vi "DriverStationGetCommands.vi"() -> ()   [LabVIEW 2019]
doc: "This VI receives instructions from the driver and manipulator controls, but only in certain robot modes. Specifically, these instructions are received while the robot is either \"running autonomously\" or in Super Test Mode. In all other robot modes, no instructions are received via the driver station. Instead they are output by the Autonomous Sequencer or completely disabled."
uses:
  refnums.vi
  dscommands.vi
  <vilib>/Rock Robotics/Network Tables/NT Read Boolean Array.vi
  dsdata.vi
  GRNF_Joystick.vi
  <vilib>/Rock Robotics/Network Tables/NT Read Boolean.vi
panel:
  in  "Buttons":bool[](array[boolean])=[FALSE, FALSE, FALSE, FALSE, FALSE, FALSE, FALSE, FALSE, FALSE, FALSE]
  in  "Right Trigger":dbl(slide) min=0.0 max=1.0 scale=0.0..1.0
  in  "Left Trigger":dbl(slide) min=0.0 max=1.0 step=0.1 scale=0.0..1.0
  in  "Right Joystick X":dbl(slide) scale=-1.0..1.0
  in  "Enable Joystick Control Override":bool
  in  "Joystick Left X":dbl(slide) scale=-1.0..1.0
  in  "Joystick Left Y":dbl(slide) scale=1.0..-1.0
  in  "Joystick Right Y":dbl(slide) scale=1.0..-1.0
  # "Left Thumbstick"
  # "Right Thumbstick"
  # "Driver A"
  # "Driver B"
  # "Driver X"
  # "Driver Y"
  # "Driver Left Bumper"
  # "Driver Right Bumper"
  # "Driver View"
  # "Driver Menu"
  # "Driver Left Joystick Button"
  # "Driver Right Joystick Button"
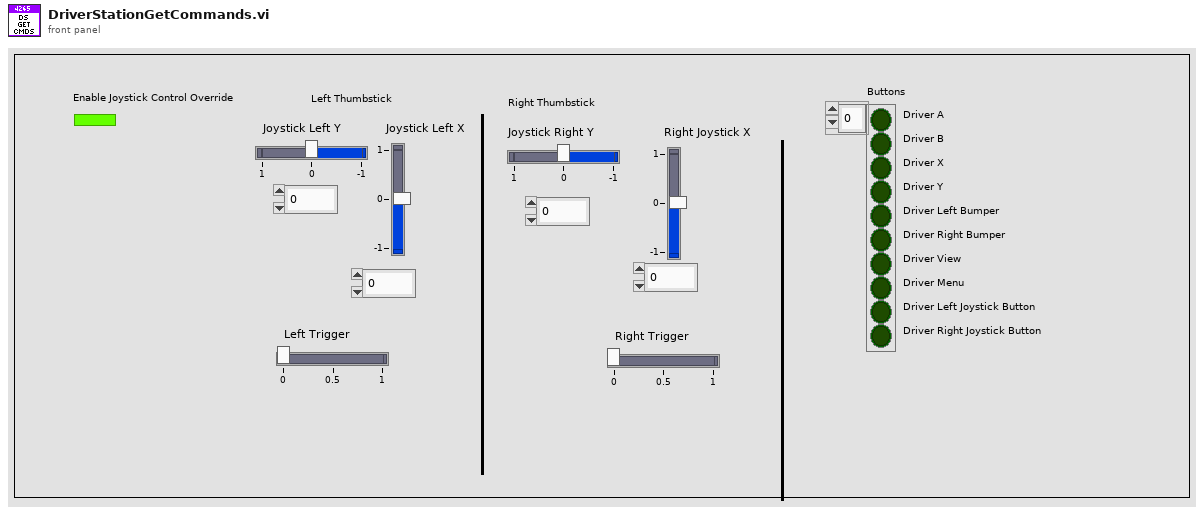
[diagram p1: front panel]
types:
  T1 = typedef "WPI_JoystickDevRef.ctl" = cluster{"Device":T2}
  T2 = typedef "WPI_JoystickDeviceEnum.ctl" = enum16{"USB 0", "USB 1", "USB 2", "USB 3", "USB 4", "USB 5"}
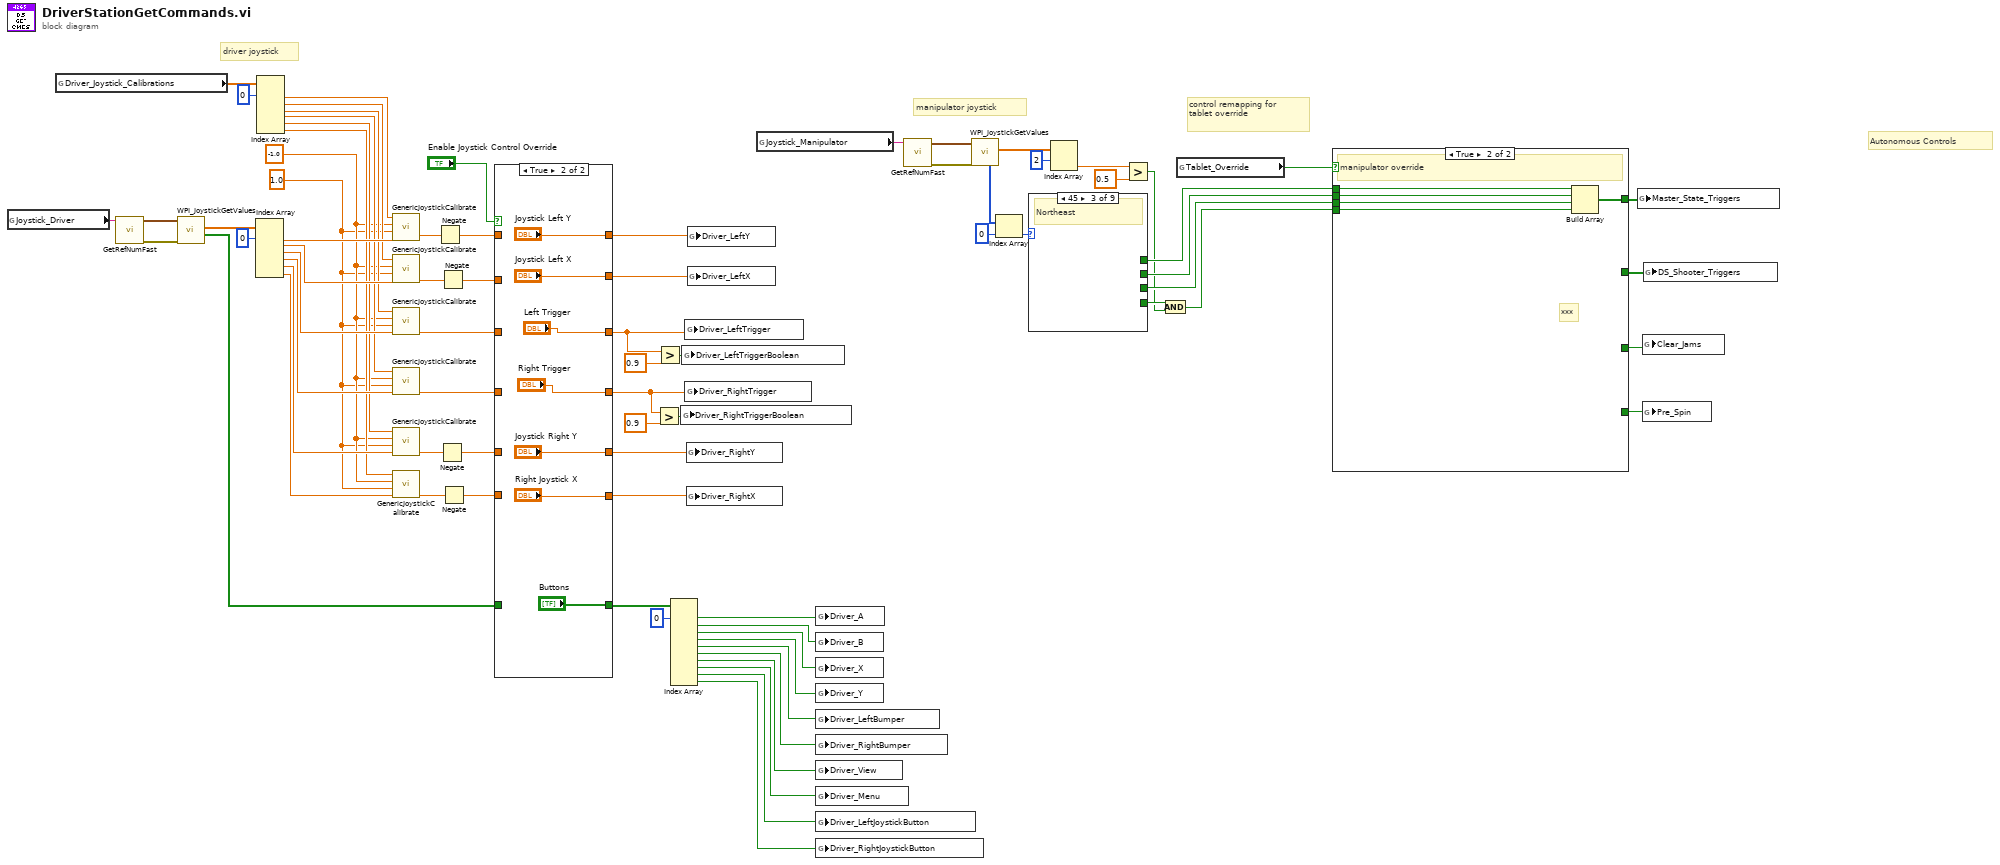
[diagram p0: block diagram]
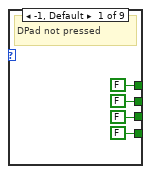
[diagram p3: hidden frame]
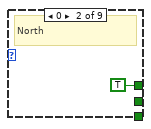
[diagram p4: hidden frame]
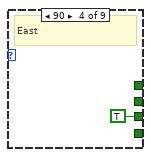
[diagram p5: hidden frame]
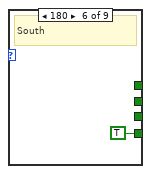
[diagram p7: hidden frame]
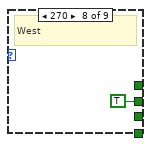
[diagram p9: hidden frame]
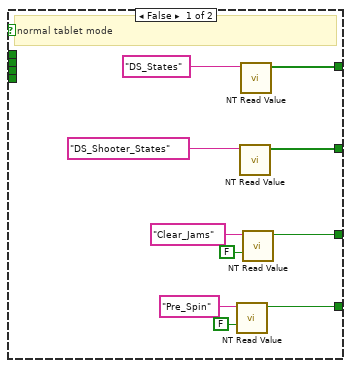
[diagram p11: hidden frame]
diagram:
  w22 = 1.0
  w23 = -1.0
  # "Autonomous Controls"
  # "control remapping for\ntablet override"
  # "manipulator joystick"
  # "driver joystick"
  n1 = global read "refnums.vi" "Joystick_Driver"() -> (w46:string)
  n2 = global read "dsdata.vi" "Driver_Joystick_Calibrations"() -> (w40:dbl[])
  n3 = call-poly "GetRefNumFast.vi"("RefNum Name"=w46) -> ("Error"=w47:errorcluster, "Device Reference"=w48:T1)  [unwired: 5 in]
  n4 = call <vilib>:"WPI_JoystickGetValues.vi"("error in (no error)"=w47, "JoystickDevRef"=w48) -> ("Buttons"=w4:bool[], "Axes"=w76:dbl[])  [unwired: 5 in, 3 out]
  n5 = Index Array(array=w76, index #1=0 ("index")) -> (element #1=w35:dbl, element #2=w34:dbl, element #3=w30:dbl, element #4=w31:dbl, element #5=w32:dbl, element #6=w33:dbl)  [unwired: 5 in]
  n6 = Index Array(array=w40, index #1=0 ("index")) -> (element #1=w24:dbl, element #2=w25:dbl, element #3=w26:dbl, element #4=w27:dbl, element #5=w28:dbl, element #6=w29:dbl)  [unwired: 5 in]
  n7 = call "GenericJoystickCalibrate.vi"("Raw Joystick Value"=w35, "Maximum"=w22, "Minimum"=w23, "Deadband"=w24) -> ("Scaled Joystick Value"=w39:dbl)  [unwired: 3 in]
  n8 = call "GenericJoystickCalibrate.vi"("Raw Joystick Value"=w34, "Maximum"=w22, "Minimum"=w23, "Deadband"=w25) -> ("Scaled Joystick Value"=w38:dbl)  [unwired: 3 in]
  n9 = call "GenericJoystickCalibrate.vi"("Raw Joystick Value"=w30, "Maximum"=w22, "Minimum"=w23, "Deadband"=w26) -> ("Scaled Joystick Value"=w16:dbl)  [unwired: 3 in]
  n10 = call "GenericJoystickCalibrate.vi"("Raw Joystick Value"=w31, "Maximum"=w22, "Minimum"=w23, "Deadband"=w27) -> ("Scaled Joystick Value"=w10:dbl)  [unwired: 3 in]
  n11 = call "GenericJoystickCalibrate.vi"("Raw Joystick Value"=w32, "Maximum"=w22, "Minimum"=w23, "Deadband"=w28) -> ("Scaled Joystick Value"=w37:dbl)  [unwired: 3 in]
  n12 = call "GenericJoystickCalibrate.vi"("Raw Joystick Value"=w33, "Maximum"=w22, "Minimum"=w23, "Deadband"=w29) -> ("Scaled Joystick Value"=w36:dbl)  [unwired: 3 in]
  n13 = Negate(x=w39) -> (-x=w19:dbl)
  n14 = Negate(x=w37) -> (-x=w7:dbl)
  n15 = Negate(x=w38) -> (-x=w18:dbl)
  n16 = Negate(x=w36) -> (-x=w6:dbl)
  n17 = case shown="True" "Enable Joystick Control Override" {
    tunnel: w16 -> [w81 _]
    tunnel: [w83 "Joystick Left Y"] -> w20
    tunnel: w19 -> [w83 _]
    tunnel: [w82 "Joystick Left X"] -> w17
    tunnel: w18 -> [w82 _]
    tunnel: [w81 "Left Trigger"] -> w11
    tunnel: w10 -> [w80 _]
    tunnel: [w80 "Right Trigger"] -> w9
    tunnel: [w79 "Joystick Right Y"] -> w8
    tunnel: w7 -> [w79 _]
    tunnel: [w78 "Right Joystick X"] -> w5
    tunnel: w6 -> [w78 _]
    tunnel: w4 -> [w77 _]
    tunnel: [w77 "Buttons"] -> w3
    frame False {
    }
    frame True {
    }
  }
  n18 = Greater?(x=w9, y=0.9) -> (0:w13:bool)
  n19 = Greater?(x=w11, y=0.9) -> (0:w12:bool)
  n20 = Index Array(array=w3, index #1=0 ("index")) -> (element #1=w73:bool, element #2=w72:bool, element #3=w71:bool, element #4=w70:bool, element #5=w69:bool, element #6=w68:bool, element #7=w67:bool, element #8=w66:bool, element #9=w65:bool, element #10=w64:bool)  [unwired: 9 in]
  n21 = global write "dscommands.vi" "Driver_RightTriggerBoolean"(w13) -> ()
  n22 = global write "dscommands.vi" "Driver_LeftTriggerBoolean"(w12) -> ()
  n23 = global write "dscommands.vi" "Driver_LeftTrigger"(w11) -> ()
  n24 = global write "dscommands.vi" "Driver_RightTrigger"(w9) -> ()
  n25 = global write "dscommands.vi" "Driver_RightY"(w8) -> ()
  n26 = global write "dscommands.vi" "Driver_RightX"(w5) -> ()
  n27 = global write "dscommands.vi" "Driver_LeftY"(w20) -> ()
  n28 = global write "dscommands.vi" "Driver_LeftX"(w17) -> ()
  n29 = global read "refnums.vi" "Joystick_Manipulator"() -> (w43:string)
  n30 = global write "dscommands.vi" "Driver_A"(w73) -> ()
  n31 = global write "dscommands.vi" "Driver_B"(w72) -> ()
  n32 = global write "dscommands.vi" "Driver_X"(w71) -> ()
  n33 = global write "dscommands.vi" "Driver_Y"(w70) -> ()
  n34 = global write "dscommands.vi" "Driver_LeftBumper"(w69) -> ()
  n35 = global write "dscommands.vi" "Driver_RightBumper"(w68) -> ()
  n36 = global write "dscommands.vi" "Driver_View"(w67) -> ()
  n37 = global write "dscommands.vi" "Driver_Menu"(w66) -> ()
  n38 = global write "dscommands.vi" "Driver_LeftJoystickButton"(w65) -> ()
  n39 = global write "dscommands.vi" "Driver_RightJoystickButton"(w64) -> ()
  n40 = call-poly "GetRefNumFast.vi"("RefNum Name"=w43) -> ("Error"=w44:errorcluster, "Device Reference"=w45:T1)  [unwired: 5 in]
  n41 = call <vilib>:"WPI_JoystickGetValues.vi"("error in (no error)"=w44, "JoystickDevRef"=w45) -> ("Axes"=w63:dbl[], "POVs"=w56:i16[])  [unwired: 5 in, 3 out]
  n42 = Index Array(array=w56, index=0) -> (element=w57:i16)
  n43 = case shown="45" w57 {
    tunnel: [FALSE TRUE _ _ _ _ _ _ _] -> w55
    tunnel: [FALSE _ _ _ _ _ _ TRUE _] -> w54
    tunnel: [FALSE _ _ TRUE _ _ _ _ _] -> w53
    tunnel: [FALSE _ _ _ _ TRUE _ _ _] -> w52
    frame -1, Default {
      # "DPad not pressed"
    }
    frame 0 {
      # "North"
    }
    frame 45 {
      # "Northeast"
    }
    frame 90 {
      # "East"
    }
    frame 135 {
      # "Southeast"
    }
    frame 180 {
      # "South"
    }
    frame 225 {
      # "Southwest"
    }
    frame 270 {
      # "West"
    }
    frame 315 {
      # "Northwest"
    }
  }
  n44 = Index Array(array=w63, index #1=2 ("index")) -> (element #2=w61:dbl)  [unwired: 1 in, 1 out]
  n45 = Greater?(x=w61, y=0.5) -> (0:w50:bool)
  n46 = And(x=w52, y=w50) -> (x .and. y?=w51:bool)
  n47 = global read "dsdata.vi" "Tablet_Override"() -> (w49:bool)
  n48 = case shown="True" w49 {
    tunnel: [w107 w113] -> w59
    tunnel: w55 -> [_ w112]
    tunnel: w54 -> [_ w111]
    tunnel: w53 -> [_ w110]
    tunnel: w51 -> [_ w109]
    tunnel: [w104 _] -> w42
    tunnel: [w101 _] -> w2
    tunnel: [w99 _] -> w1
    frame False {
      # "normal tablet mode"
      n49 = call-poly <vilib>:"NT Read Value.vi"("Default Value"=FALSE, "Name"="Pre_Spin" ("refnum name")) -> ("Boolean"=w101:bool)  [unwired: 8 in, 1 out]
      n50 = call-poly <vilib>:"NT Read Value.vi"("Name"="DS_Shooter_States" ("refnum name")) -> ("Boolean Array"=w99:bool[])  [unwired: 9 in, 1 out]
      n51 = call-poly <vilib>:"NT Read Value.vi"("Name"="DS_States" ("refnum name")) -> ("Boolean Array"=w107:bool[])  [unwired: 9 in, 1 out]
      n52 = call-poly <vilib>:"NT Read Value.vi"("Default Value"=FALSE, "Name"="Clear_Jams" ("refnum name")) -> ("Boolean"=w104:bool)  [unwired: 8 in, 1 out]
    }
    frame True {
      # "***"
      # "manipulator override"
      n53 = Build Array(w112, w111, w110, w109) -> (w113:bool[])
    }
  }
  n54 = global write "dscommands.vi" "Master_State_Triggers"(w59) -> ()
  n55 = global write "dscommands.vi" "Clear_Jams"(w42) -> ()
  n56 = global write "dscommands.vi" "Pre_Spin"(w2) -> ()
  n57 = global write "dscommands.vi" "DS_Shooter_Triggers"(w1) -> ()
